vi "2ndOrderDerivate.vi"(8 "t_capture":dbl format="%0.2f", 9 "initial condition":dbl format="%0.2f", 10 "x":dbl format="%0.2f", 11 "Utilities in":refnum<class "Utilities.lvclass">) -> (0 "error out":errorcluster, 1 "debug_dt":dbl[](array[numeric]), 2 "dx/dt":dbl format="%0.2f", 3 "Utilities out":refnum<class "Utilities.lvclass">)   [LabVIEW 2023, in "Utilities.lvclass"]
uses:
  Utilities.lvclass
  <vilib>/Analysis/NI_AALPro.lvlib
panel:
  in  "initialize":bool
  in  "dt":dbl=1.0 format="%0.2f"
  out "error":i32
  in  "error in (no error)":errorcluster
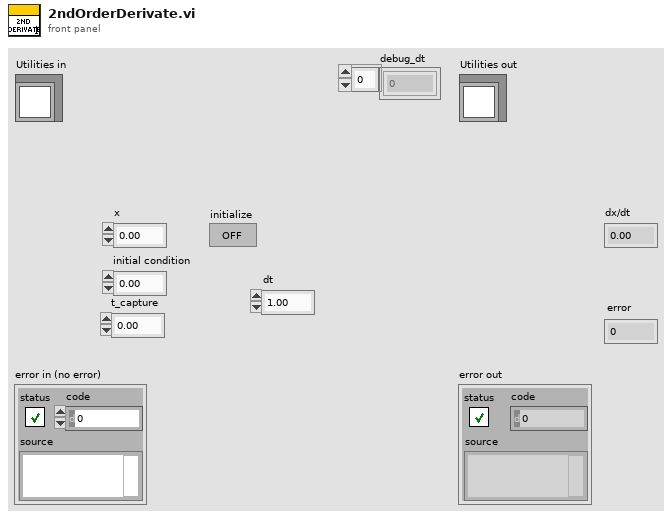
[diagram p1: front panel]
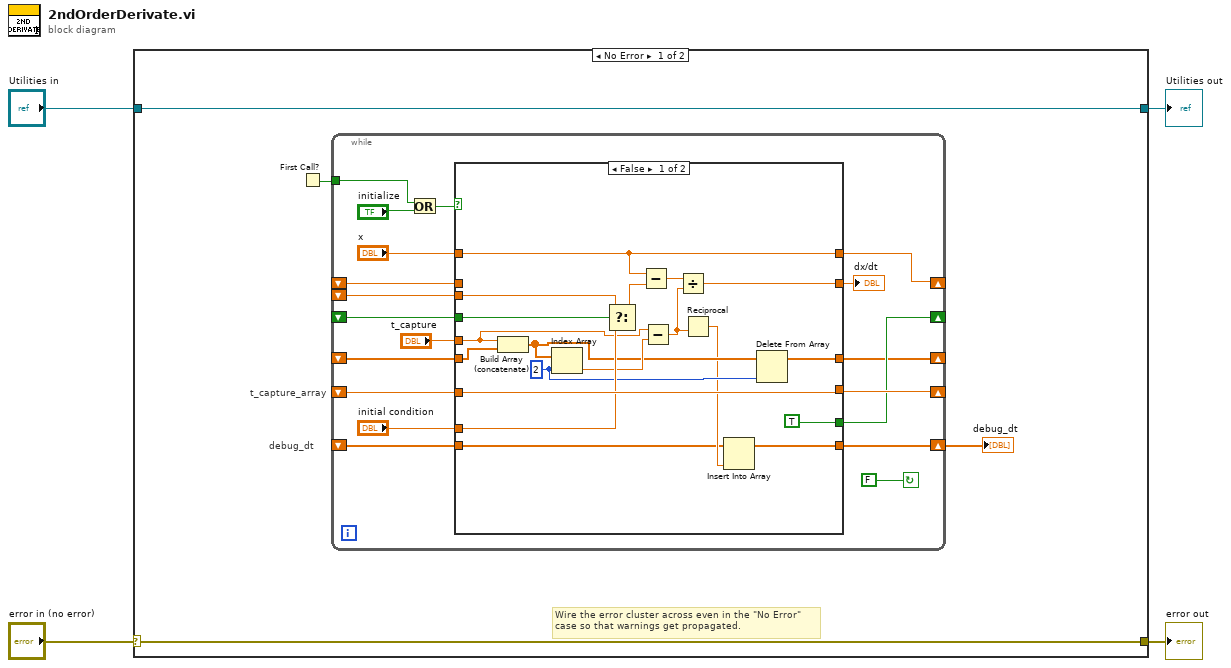
[diagram p0: block diagram]
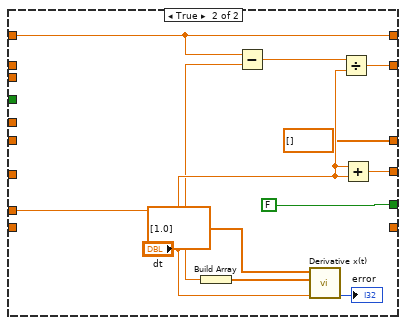
[diagram p2: hidden frame]
diagram:
  n1 = case shown="No Error" "error in (no error)" {
    selector: "error in (no error)" -> [w7 w59]
    tunnel: [w7 w59] -> w3
    tunnel: [w8 w58] -> w1
    tunnel: "Utilities in" -> [w8 w58]
    frame No Error {
      # "debug_dt"
      # "t_capture_array"
      # "Wire the error cluster across even in the \"No Error\"\ncase so that warnings get propagated."
      n2 = First Call?() -> (First Call?: T/F=w6:bool)
      n3 = while {
        shift-left: _ -> [w16]
        shift-right: [w17] -> _
        shift-left: _ -> [w20]
        shift-right: [w23] -> _
        tunnel: w6 -> [w26]
        shift-left: _ -> [w19]
        shift-left: _ -> [w15]
        shift-right: [w18] -> _
        shift-right: [w12] -> _
        shift-left: _ -> [w11]
        shift-right: [w10] -> w5
        shift-left: _ -> [w9]
        stop <- FALSE continue-if-true
        n4 = Or(x=w26, y="initialize") -> (x .or. y?=w24:bool)
        n5 = case shown="False" w24 {
          tunnel: [w44 w53] -> w23
          tunnel: "x" -> [w45 w55]
          tunnel: [w46 w56] -> w21
          tunnel: w20 -> [w44 _]
          tunnel: w19 -> [w40 _]
          tunnel: [w45 w55] -> w18
          tunnel: [TRUE FALSE] -> w17
          tunnel: w16 -> [w41 _]
          tunnel: w15 -> [_ _]
          tunnel: "initial condition" -> [w39 w49]
          tunnel: "t_capture" -> [w37 _]
          tunnel: [w33 dbl[] []] -> w12
          tunnel: w11 -> [w32 _]
          tunnel: [w29 _] -> w10
          tunnel: w9 -> [w28 _]
          frame False {
            w34 = 2 ("index")
            n6 = Build Array (concatenate)(w37, w32) -> (w35:dbl[])
            n7 = Index Array(array=w35, index=w34) -> (element=w36:dbl)
            n8 = Select(t=w40, s=w41, f=w39) -> (s? t:f=w38:dbl)
            n9 = Subtract(x=w45, y=w38) -> (x-y=w42:dbl)
            n10 = Subtract(x=w37, y=w36) -> (x-y=w31:dbl)
            n11 = Divide(x=w42, y=w31) -> (x/y=w46:dbl)
            n12 = Reciprocal(x=w31) -> (1/x=w30:dbl)
            n13 = Insert Into Array(array=w28, new element=w30) -> (w29:dbl[])  [unwired: 1 in]
            n14 = Delete From Array(array=w35, index=w34) -> (array with subset deleted=w33:dbl[])  [unwired: 1 in, 1 out]
          }
          frame True {
            n15 = Build Array(w49) -> (w48:dbl[])
            n16 = Subtract(x=w55, y=w49) -> (x-y=w57:dbl)
            n17 = call <vilib>:"Derivative x(t).vi"("dt"="dt", "Initial Condition"=w48, "X"=dbl[] [1.0]) -> ("error"=→"error":i32)  [unwired: 7 in, 1 out]
            n18 = Divide(x=w57, y="dt") -> (x/y=w56:dbl)
            n19 = Add(x="dt", y="dt") -> (x+y=w53:dbl)
          }
        }
        "dx/dt" <- w21
      }
      "debug_dt" <- w5
    }
    frame Error {
    }
  }
  "error out" <- w3
  "Utilities out" <- w1
